vi "globalConstants.vi"() -> ()   [LabVIEW 2017]
panel:
  in  "moduleOpenPosition2":u32=500 min=1
  in  "moduleClosePosition2":u32=83 min=1
  in  "moduleOpenPosition":u32=403 min=1
  in  "moduleClosePosition":u32=8 min=1
  in  "menuOpenPosition":u32=80 min=1
  in  "menuClosePosition":u32=1 min=1
  in  "logoOpenPosition":u32=80 min=1
  in  "logoClosePosition":u32=17 min=1
  out "StartProfileTCL":string="StartProfile"
  out "CleanupUIMHL":string="CleanupUI"
  out "ShutdownSuccess":string="Shutdown successful."
  out "InitShutdownSuccess":string="Initiating shutdown..."
  out "InitShutdownFail":string="An error occurred when attempting to shutdown. Check ErrorLog.txt for more detail."
  out "ResetFail":string="An error occurred when attempting to reset a profile. Check ErrorLog.txt for more detail."
  out "ResetSuccess":string="Thermal profile reset."
  out "LandChamberFail":string="An error occurred when attempting to land the chamber to ambient temperature. Check ErrorLog.txt for more detail."
  out "LandChamberSuccess":string="Landing chamber to ambient temperature..."
  out "StopScanFail":string="An error occured when attempting to stop a scan of one or more DAQ devices. Check ErrorLog.txt for more detail."
  out "StopScanSuccess":string="Stopped DAQ device scan."
  out "StopProfileSuccess":string="Chamber controller profile stopped."
  out "StopProfileFail":string="An error occured when attempting to stop the chamber controller profile. Check ErrorLog.txt for more detail."
  out "ProfileSuccess":string="Running thermal profile..."
  out "ProfileFail":string="An error occurred when attempting to start a profile. Check ErrorLog.txt for more detail."
  out "SingleScanFail":string="An error occured when attempting to scan one or more DAQ devices. Check ErrorLog.txt for more detail."
  out "SingleScanSuccess":string="Single scan completed succesfully."
  out "ControllerNotInit":string="An error occurred when attempting to initialize the chamber controller. Check ErrorLog.txt for more detail."
  out "ControllerInit":string="Chamber controller initialized successfully."
  out "DAQNotInit":string="An error occurred when attempting to initialize one or more DAQ devices. Check ErrorLog.txt for more detail."
  out "CleanupMHL":string="Cleanup"
  out "InitUIMHL":string="InitUI"
  out "GetUIRefsMHL":string="GetUIRefs"
  out "OpenDataLog":string="OpenDataLog"
  out "GetUIRefsCCL":string="GetUIRefs"
  out "InitUICCL":string="InitUI"
  out "CloseControllerRef":string="CloseControllerRef"
  out "CleanupCCL":string="Cleanup"
  out "InitExitTML":string="InitExit"
  out "GetUIRefsTML":string="GetUIRefs"
  out "InitUITML":string="InitUI"
  out "CleanupTML":string="Cleanup"
  out "CloseDataLog":string="CloseDataLog"
  out "CloseDeviceRef":string="CloseDeviceRef"
  out "UpdateTMLData":string="UpdateTMLData"
  out "UpdateCCLData":string="UpdateCCLData"
  out "GetUIRefsTCL":string="GetUIRefs"
  out "InitUITCL":string="InitUI"
  out "UpdateTCLData":string="UpdateTCLData"
  out "CleanupTCL":string="Cleanup"
  out "InitExitTCL":string="InitExit"
  out "InitExitCCL":string="InitExit"
  out "StopScan":string="StopScan"
  out "WaitOnCCLExit":string="WaitOnCCLExit"
  out "WaitOnTCLExit":string="WaitOnTCLExit"
  out "WaitOnTMLExit":string="WaitOnTMLExit"
  out "InitExit":string="InitExit"
  out "UpdateDisplayTML":string="UpdateDisplay"
  out "UpdateDisplayCCL":string="UpdateDisplay"
  out "UpdateDisplayTCL":string="UpdateDisplay"
  out "ResetTCL":string="Reset"
  out "RampChamberCCL":string="RampChamber"
  out "ReturnToAmbientTCL":string="ReturnToAmbient"
  out "FPInitialized":string="Front panel initialized."
  out "InitProcesses":string="InitProcesses"
  out "ExitTCL":string="Exit"
  out "TempScanConfigured":string="Temperature scan configured."
  out "GetTempData":string="GetTempData"
  out "SetDwell":string="SetDwell"
  out "InitTCL":string="Init"
  out "SetTempState":string="SetTempState"
  out "RampChamberTCL":string="RampChamber"
  out "SetCycles":string="SetCycles"
  out "CheckDwell":string="CheckDwell"
  out "CheckRange":string="CheckRange"
  out "SingleScanTML":string="SingleScan"
  out "Error in CCL":string="Error occured in chamber controller loop. Check Error Log.txt for more detail."
  out "Temp Logging Started":string="Temperature logging started."
  out "Temp Monitors Configured":string="Temperature monitors configured for scanning."
  out "ContinuousScan":string="ContinuousScan"
  out "Timestamp in seconds":string="%s %<%m.%d.%y %I.%M.%S %p>T"
  out "Error in TML":string="Error occured in temperature monitor loop. Check Error Log.txt for more detail."
  out "ErrorMHL":string="Error"
  out "DAQInit":string="DAQ devices initialized successfully."
  out "InitDAQDevices":string="InitDAQDevices"
  out "InitController":string="InitController"
  out "InitializeDevices":string="InitializeDevices"
  out "ReturnToAmbientMHL":string="ReturnToAmbient"
  out "ThermalCycle":string="ThermalCycle"
  out "SingleScanMHL":string="SingleScan"
  out "ExitCCL":string="Exit"
  out "ExitTML":string="Exit"
  out "Temp Log":string="Temp Log"
  out "InitCCL":string="Init"
  out "InitTML":string="Init"
  out "UpdateDisplayMHL":string="UpdateDisplay"
  out "ExitMHL":string="Exit"
  out "InitMHL":string="Init"
  # "Queue Messages"
  # "MHL Queue"
  # "TML Queue"
  # "CCL Queue"
  # "TCL Queue"
  # "Status Messages"
  # "MHL Queue"
  # "TML Queue"
  # "TCL Queue"
  # "CCL Queue"
  # "Configuration"
  # "Timestamp in seconds"
  # "UI Settings"
  # "Splitters"
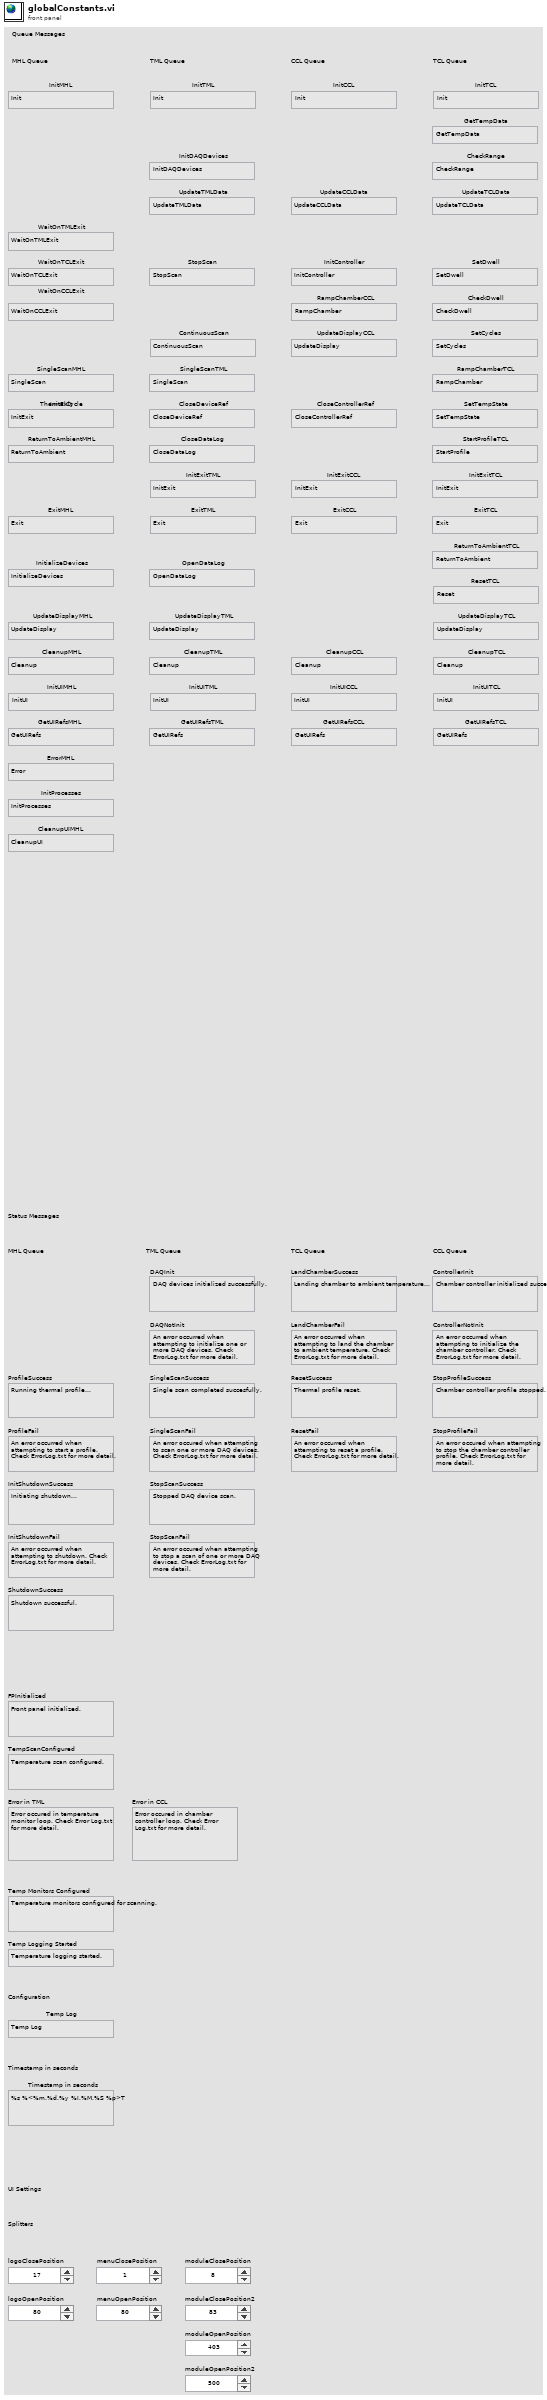
[diagram p1: front panel]
diagram:
